vi "configureAcquisition.vi"(0 "HGF_IMAQDevice":refnum<class "HGF_IMAQDevice.lvclass">, 2 "Continuous?":enum16{"One-Shot", "Continuous"}(ring)=enum."Continuous", 3 "Number of buffers":u32, 5 "error in (no error)":errorcluster, 6 "Region of Interest":i32[](array[numeric]), 7 "Memory Location":enum16{"System", "Onboard"}(ring), 8 "Buffer Parameters":cluster{"Skip Count":u32, "Channel":i32}[](array[cluster]), 9 "Image Array":T1[](array[typedef])) -> (14 "dup HGF_IMAQDevice":refnum<class "HGF_IMAQDevice.lvclass">, 19 "error out":errorcluster)   [LabVIEW 2014, in "HGF_IMAQ.lvlib" / "HGF_IMAQDevice.lvclass"]
doc: "Configures a low-level acquisition previously opened with IMAQdx Open Camera VI. Specify the acquisition type with the Continuous? and Number of Buffers parameters. \n\nSnap: Continuous = 0; Buffer Count = 1 \nSequence: Continuous = 0; Buffer Count > 1 \nGrab: Continuous = 1; Buffer Count > 1"
uses:
  HGF_IMAQDevice.lvclass
  <vilib>/vision/Image Controls.llb/IMAQ Image.ctl
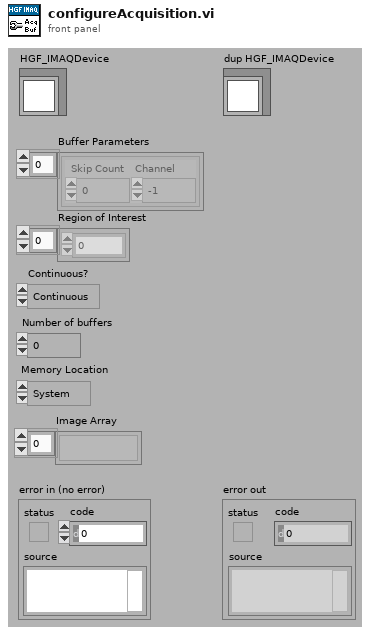
[diagram p1: front panel]
types:
  T1 = typedef "IMAQ Image.ctl" = refnum<image>
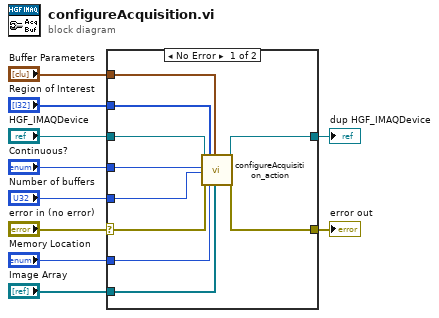
[diagram p0: block diagram]
diagram:
  n1 = case shown="No Error" "error in (no error)" {
    selector: "error in (no error)" -> [w20 w22]
    tunnel: [w19 w22] -> w9
    tunnel: [w17 w21] -> w7
    tunnel: "HGF_IMAQDevice" -> [w18 w21]
    tunnel: "Continuous?" -> [w16 _]
    tunnel: "Region of Interest" -> [w15 _]
    tunnel: "Buffer Parameters" -> [w14 _]
    tunnel: "Number of buffers" -> [w13 _]
    tunnel: "Image Array" -> [w11 _]
    tunnel: "Memory Location" -> [w12 _]
    frame No Error {
      n2 = call-dynamic "configureAcquisition_action.vi"("HGF_IMAQDevice"=w18, "Continuous?"=w16, "Number of buffers"=w13, "error in (no error)"=w20, "Region of Interest"=w15, "Memory Location"=w12, "Buffer Parameters"=w14, "Image Array"=w11) -> ("dup HGF_IMAQDevice"=w17:refnum<class "HGF_IMAQDevice.lvclass">, "error out"=w19:errorcluster)  [unwired: 10 in]
    }
    frame Error {
    }
  }
  "error out" <- w9
  "dup HGF_IMAQDevice" <- w7
